vi "Servo_Initialization(SubVI).vi"(7 "error in (no error)":errorcluster, 10 "refnum":T1) -> (0 "error out":errorcluster, 2 "output cluster":T2, 3 "refnum out":T1)   [LabVIEW 2017]
uses:
  <vilib>/Utility/config.llb/Config Data RefNum.ctl
  <vilib>/Utility/config.llb/Read Key (Double).vi
  <vilib>/Utility/config.llb/NI_LVConfig.lvlib
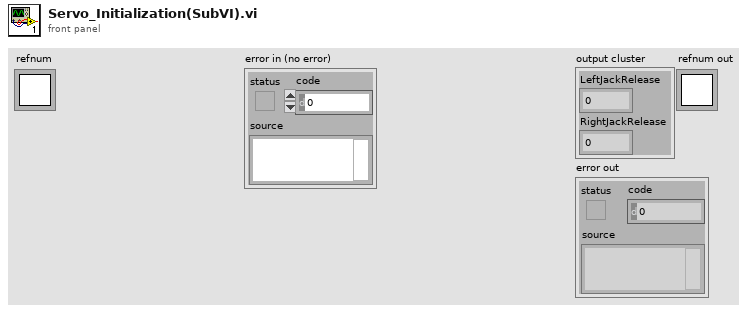
[diagram p1: front panel]
types:
  T1 = typedef "NI_LVConfig.lvlib/Config Data RefNum.ctl" = refnum<k1>
  T2 = cluster{"LeftJackRelease":dbl, "RightJackRelease":dbl}
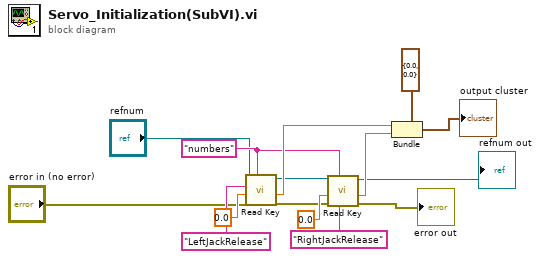
[diagram p0: block diagram]
diagram:
  w8 = "numbers" ("section")
  n1 = call-poly <vilib>:"Read Key.vi"("section"=w8, "error in (no error)"="error in (no error)", "default value"=0.0, "key"="LeftJackRelease", "refnum"="refnum") -> ("error out"=w6:errorcluster, "value"=w14:dbl, "refnum out"=w7:T1)  [unwired: 3 in, 1 out]
  n2 = call-poly <vilib>:"Read Key.vi"("section"=w8, "error in (no error)"=w6, "default value"=0.0, "key"="RightJackRelease", "refnum"=w7) -> ("error out"=→"error out":errorcluster, "value"=w15:dbl, "refnum out"=→"refnum out":T1)  [unwired: 3 in, 1 out]
  n3 = Bundle(cluster=T2 {"LeftJackRelease"=0.0, "RightJackRelease"=0.0} ("Servo Values"), "LeftJackRelease"=w14, "RightJackRelease"=w15) -> (→"output cluster":T2)
